vi "BTK Model_Janson.vi"(9 "V":dbl[](array[numeric])=[-0.1, -0.099, -0.098, -0.097, -0.096, -0.095, -0.094, -0.093, -0.092, -0.091, -0.09000000000000001, -0.08900000000000001, -0.08800000000000001, -0.08700000000000001, -0.08600000000000001, -0.085, -0.084, -0.083, -0.082, -0.081, -0.08, -0.079, -0.07800000000000001, -0.07700000000000001, -0.07600000000000001, -0.07500000000000001, -0.07400000000000001, -0.07300000000000001, -0.07200000000000001, -0.07100000000000001, -0.07, -0.069, -0.068, -0.067, -0.066, -0.065, -0.064, -0.063, -0.062000000000000006, -0.061000000000000006, -0.060000000000000005, -0.059000000000000004, -0.058, -0.057, -0.05600000000000001, -0.05500000000000001, -0.054000000000000006, -0.053000000000000005, -0.052000000000000005, -0.051000000000000004, -0.05, -0.049, -0.048, -0.04700000000000001, -0.046000000000000006, -0.045000000000000005, -0.044000000000000004, -0.043000000000000003, -0.042, -0.041, -0.04000000000000001, -0.03900000000000001, -0.038000000000000006, -0.037000000000000005, -0.036000000000000004, -0.035, -0.034, -0.033, -0.032, -0.031, -0.03, -0.028999999999999998, -0.027999999999999997, -0.02700000000000001, -0.02600000000000001, -0.02500000000000001, -0.024000000000000007, -0.023000000000000007, -0.022000000000000006, -0.021000000000000005, -0.020000000000000004, -0.019000000000000003, -0.018000000000000002, -0.017, -0.016, -0.015, -0.013999999999999999, -0.012999999999999998, -0.01200000000000001, -0.01100000000000001, -0.010000000000000009, -0.009000000000000008, -0.008000000000000007, -0.007000000000000006, -0.006000000000000005, -0.0050000000000000044, -0.0040000000000000036, -0.0030000000000000027, -0.0020000000000000018, -0.0010000000000000009, 0.0, 0.0010000000000000009, 0.0020000000000000018, 0.0030000000000000027, 0.0040000000000000036, 0.0049999999999999906, 0.0059999999999999915, 0.006999999999999992, 0.007999999999999993, 0.008999999999999994, 0.009999999999999995, 0.010999999999999996, 0.011999999999999997, 0.012999999999999998, 0.013999999999999999, 0.015, 0.016, 0.017, 0.018000000000000002, 0.019000000000000003, 0.01999999999999999, 0.02099999999999999, 0.021999999999999992, 0.022999999999999993, 0.023999999999999994, 0.024999999999999994, 0.025999999999999995, 0.026999999999999996, 0.027999999999999997, 0.028999999999999998, 0.03, 0.031, 0.032, 0.033, 0.034, 0.035, 0.036000000000000004, 0.037000000000000005, 0.038000000000000006, 0.03900000000000001, 0.04000000000000001, 0.04100000000000001, 0.04200000000000001, 0.04300000000000001, 0.04400000000000001, 0.044999999999999984, 0.045999999999999985, 0.046999999999999986, 0.04799999999999999, 0.04899999999999999, 0.04999999999999999, 0.05099999999999999, 0.05199999999999999, 0.05299999999999999, 0.05399999999999999, 0.05499999999999999, 0.055999999999999994, 0.056999999999999995, 0.057999999999999996, 0.059, 0.06, 0.061, 0.062, 0.063, 0.064, 0.065, 0.066, 0.067, 0.068, 0.069, 0.07, 0.07100000000000001, 0.07200000000000001, 0.07300000000000001, 0.07400000000000001, 0.07500000000000001, 0.07599999999999998, 0.07699999999999999, 0.07799999999999999, 0.07899999999999999, 0.07999999999999999, 0.08099999999999999, 0.08199999999999999, 0.08299999999999999, 0.08399999999999999, 0.08499999999999999, 0.086, 0.087, 0.088, 0.089, 0.09, 0.091, 0.092, 0.093, 0.094, 0.095, 0.096, 0.097, 0.098, 0.099, 0.1], 10 "Parameters":T1={"Gama"=0.001, "Delta"=0.03, "Z"=1.0, "P"=0.0, "T"=50.0, "Lower limit"=-10.0, "Upper limit"=10.0, "Resolution"=0.01} {"Resolution" format="%#_6peV"; "Upper limit" format="%#_6peV"; "Lower limit" format="%#_6peV"; "T" format="%#_6pK"; "Delta" format="%#_6peV"; "Gama" format="%#_6peV"}) -> (2 "Conductivity":dbl[](array[numeric]))   [LabVIEW 2021]
uses:
  Parameters.ctl
panel:
  in  "Normalize":bool
  out "1/x":dbl
  out "I-V":cluster{"Steps":dbl[], "dX/dt":dbl[]}(graph)
  out "f(E-eV)-f(E)":cluster{"Steps":dbl[], "dX/dt":dbl[]}(graph)
  out "Z":cluster{"Steps":dbl[], "dX/dt":dbl[]}(graph)
  out "dIdV":cluster{"Steps":dbl[], "dX/dt":dbl[]}(graph)
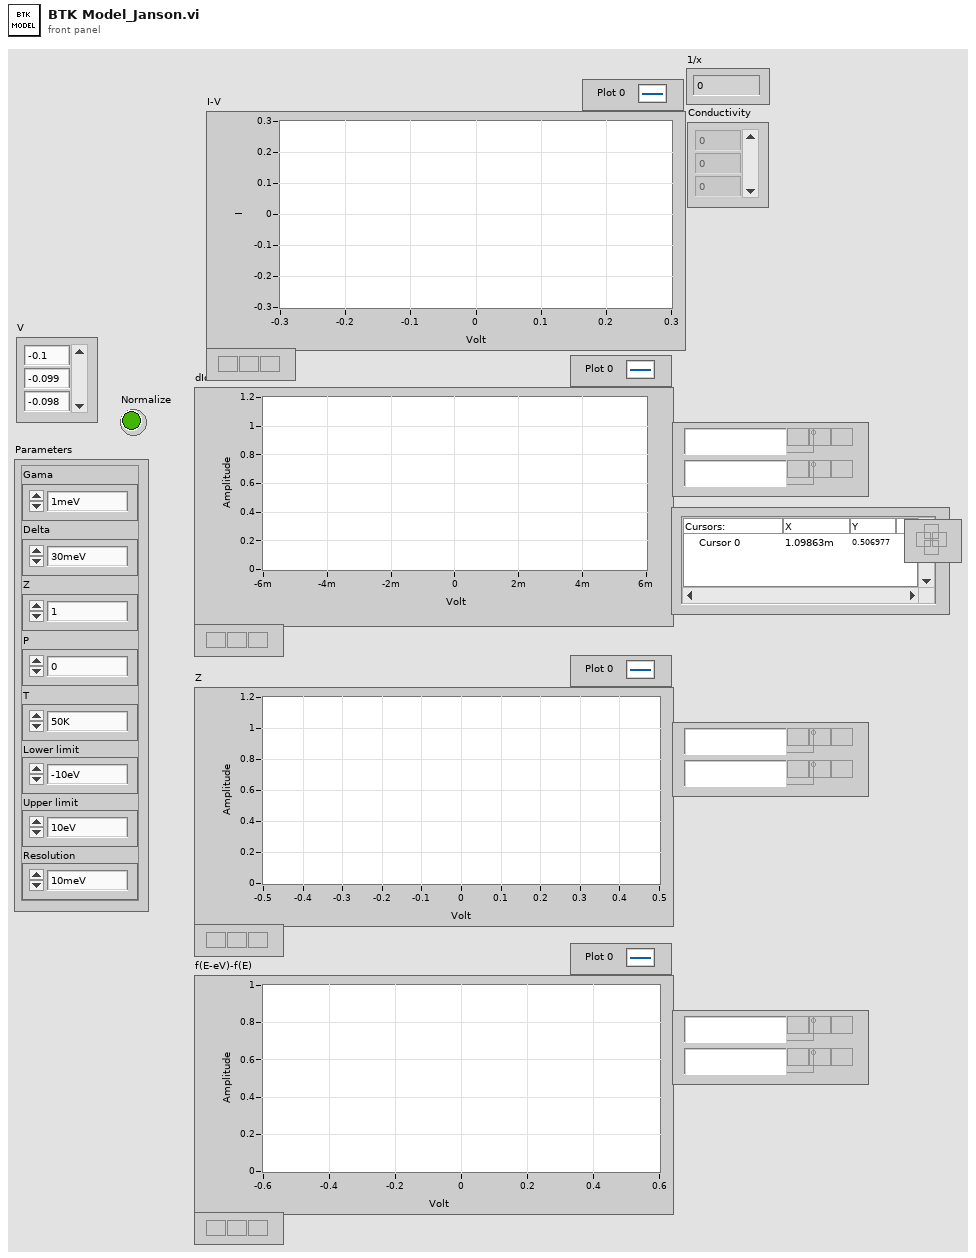
[diagram p1: front panel]
types:
  T1 = typedef "Parameters.ctl" = cluster{"Gama":dbl, "Delta":dbl, "Z":dbl, "P":dbl, "T":dbl, "Lower limit":dbl, "Upper limit":dbl, "Resolution":dbl}
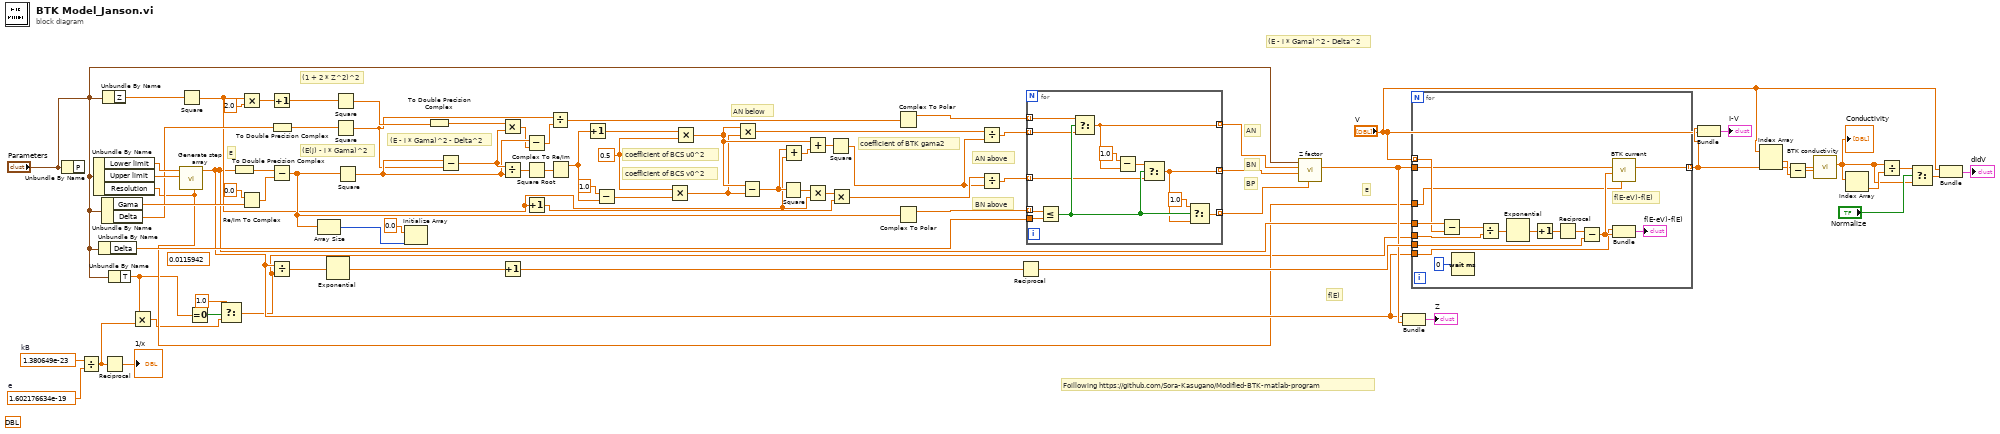
[diagram p0: block diagram]
diagram:
  w19 = 1.602176634e-19  # e
  (unwired) ext[unit] 1.602176634e-19
  w20 = 1.380649e-23  # kB
  (unwired) 0.0115942
  w66 = 0.5
  # "f(E)"
  # "E"
  # "BP"
  # "BN"
  # "AN"
  # "Foillowing https://github.com/Sora-Kasugano/Modified-BTK-matlab-program"
  # "BN above"
  # "AN above"
  # "AN below"
  # "(E(j) - i * Gama)^2"
  # "(E - i * Gama)^2 - Delta^2"
  # "(1 + 2 * Z^2)^2"
  # "E"
  # "(E - i * Gama)^2 - Delta^2"
  # "coefficient of BTK gama2"
  # "coefficient of BCS v0^2"
  # "coefficient of BCS u0^2"
  n1 = Unbundle By Name("Parameters") -> ()  [unwired: 1 out]
  n2 = Divide(x=w20, y=w19) -> (x/y=w7:dbl)
  n3 = Unbundle By Name("Parameters") -> ("Lower limit"=w80:dbl, "Upper limit"=w79:dbl, "Resolution"=w14:dbl)
  n4 = Unbundle By Name("Parameters") -> ("Delta"=w37:dbl)
  n5 = Unbundle By Name("Parameters") -> ("Gama"=w77:dbl, "Delta"=w74:dbl)
  n6 = Unbundle By Name("Parameters") -> ("Z"=w65:dbl)
  n7 = Reciprocal(x=w7) -> (1/x=→"1/x":dbl)
  n8 = Unbundle By Name("Parameters") -> ("T"=w6:dbl)
  n9 = Multiply(x=w6, y=w7) -> (x*y=w8:dbl)
  n10 = call "Generate step array.vi"("Step"=w14, "End"=w79, "Start"=w80) -> ("Steps"=w22:dbl[])  [unwired: 8 in]
  n11 = Square(x=w65) -> (x^2=w43:dbl)
  n12 = Equal To 0?(x=w6) -> (x = 0?=w11:bool)
  n13 = Select(t=1.0, s=w11, f=w8) -> (s? t:f=w9:dbl)
  n14 = To Double Precision Complex(1:w22) -> (0:w76:cdb[])
  n15 = Multiply(x=w43, y=2.0) -> (x*y=w59:dbl)
  n16 = Re/Im To Complex(1:w77, 2:0.0) -> (0:w75:cdb)
  n17 = Increment(x=w59) -> (x+1=w58:dbl)
  n18 = Subtract(x=w76, y=w75) -> (x-y=w46:cdb[])
  n19 = Divide(x=w22, y=w9) -> (x/y=w33:dbl[])
  n20 = To Double Precision Complex(1:w74) -> (0:w73:cdb)
  n21 = Array Size(array=w46) -> (size(s)=w61:i32)
  n22 = Exponential(1:w33) -> (0:w32:dbl[])
  n23 = Square(x=w58) -> (x^2=w57:dbl)
  n24 = Square(x=w73) -> (x^2=w51:cdb)
  n25 = Square(x=w46) -> (x^2=w54:cdb[])
  n26 = Initialize Array(0.0, w61) -> ()  [unwired: 1 out]
  n27 = To Double Precision Complex(1:w57) -> (0:w55:cdb)
  n28 = Subtract(x=w54, y=w51) -> (x-y=w56:cdb[])
  n29 = Multiply(x=w55, y=w56) -> (x*y=w53:cdb[])
  n30 = Divide(x=w56, y=w54) -> (x/y=w72:cdb[])
  n31 = Increment(x=w32) -> (x+1=w31:dbl[])
  n32 = Subtract(x=w54, y=w53) -> (x-y=w52:cdb[])
  n33 = Square Root(x=w72) -> (sqrt(x)=w71:cdb[])
  n34 = Increment(x=w43) -> (x+1=w41:dbl)
  n35 = Divide(x=w51, y=w52) -> (x/y=w47:cdb[])
  n36 = Complex To Re/Im(x + iy=w71) -> (x=w69:dbl[])  [unwired: 1 out]
  n37 = Increment(x=w69) -> (x+1=w70:dbl[])
  n38 = Subtract(x=1.0, y=w69) -> (x-y=w67:dbl[])
  n39 = Multiply(x=w66, y=w67) -> (x*y=w49:dbl[])
  n40 = Multiply(x=w70, y=w66) -> (x*y=w50:dbl[])
  n41 = Multiply(x=w50, y=w49) -> (x*y=w48:dbl[])
  n42 = Subtract(x=w50, y=w49) -> (x-y=w45:dbl[])
  n43 = Square(x=w45) -> (x^2=w44:dbl[])
  n44 = Add(x=w45, y=w43) -> (x+y=w64:dbl[])
  n45 = Add(x=w50, y=w64) -> (x+y=w63:dbl[])
  n46 = Multiply(x=w44, y=w43) -> (x*y=w42:dbl[])
  n47 = Square(x=w63) -> (x^2=w39:dbl[])
  n48 = Multiply(x=w42, y=w41) -> (x*y=w40:dbl[])
  n49 = Complex To Polar(r * e^(i*theta)=w47) -> (r=w36:dbl[])  [unwired: 1 out]
  n50 = Complex To Polar(r * e^(i*theta)=w46) -> (r=w38:dbl[])  [unwired: 1 out]
  n51 = Divide(x=w48, y=w39) -> (x/y=w34:dbl[])
  n52 = Divide(x=w40, y=w39) -> (x/y=w35:dbl[])
  n53 = Reciprocal(x=w31) -> (1/x=w30:dbl[])
  n54 = for {
    tunnel: w38 -> [w87] mode=indexing
    tunnel: w37 -> [w88]
    tunnel: w36 -> [w86] mode=indexing
    tunnel: w35 -> [w85] mode=indexing
    tunnel: w34 -> [w84] mode=indexing
    tunnel: [w83] -> w28 mode=indexing
    tunnel: [w82] -> w27 mode=indexing
    tunnel: [w81] -> w26 mode=indexing
    n55 = Less Or Equal?(x=w87, y=w88) -> (x <= y?=w89:bool)
    n56 = Select(t=w86, s=w89, f=w84) -> (s? t:f=w83:dbl)
    n57 = Subtract(x=1.0, y=w83) -> (x-y=w92:dbl)
    n58 = Select(t=w92, s=w89, f=w85) -> (s? t:f=w82:dbl)
    n59 = Select(t=1.0, s=w89, f=w82) -> (s? t:f=w81:dbl)
  }
  n60 = call "Z factor.vi"("BP"=w26, "BN"=w27, "AN"=w28, "Parameters"="Parameters") -> ("z factor"=w24:dbl[])  [unwired: 7 in]
  n61 = Bundle("Steps"=w22, "z factor"=w24) -> (→"Z":cluster{"Steps":dbl[], "z factor":dbl[]})  [unwired: 1 in]
  n62 = for {
    tunnel: "V" -> [w107] mode=indexing
    tunnel: w22 -> [w108]
    tunnel: w9 -> [w104]
    tunnel: w30 -> [w102]
    tunnel: w24 -> [w99]
    tunnel: [w98] -> w13 mode=indexing
    tunnel: w22 -> [w94]
    tunnel: w14 -> [w93]
    # "f(E-eV)-f(E)"
    n63 = Subtract(x=w108, y=w107) -> (x-y=w106:dbl[])
    n64 = Wait (ms)(milliseconds to wait=u32 0) -> ()  [unwired: 1 out]
    n65 = Divide(x=w106, y=w104) -> (x/y=w105:dbl[])
    n66 = Exponential(1:w105) -> (0:w103:dbl[])
    n67 = Increment(x=w103) -> (x+1=w101:dbl[])
    n68 = Reciprocal(x=w101) -> (1/x=w100:dbl[])
    n69 = Subtract(x=w100, y=w102) -> (x-y=w97:dbl[])
    n70 = call "BTK current.vi"("dx"=w93, "f factor"=w97, "z factor"=w99) -> ("I current"=w98:dbl)  [unwired: 8 in]
    n71 = Bundle("Steps"=w94, w97) -> (→"f(E-eV)-f(E)":cluster{"Steps":dbl[], dbl[]})  [unwired: 1 in]
  }
  n72 = Bundle(w13, "V"="V") -> (→"I-V":cluster{dbl[], "V":dbl[]})  [unwired: 1 in]
  n73 = Index Array(array="V") -> (element #1=w17:dbl, element #2=w16:dbl)  [unwired: 2 in]
  n74 = Subtract(x=w16, y=w17) -> (x-y=w15:dbl)
  n75 = call "BTK conductivity.vi"("dx"=w15, "Current"=w13) -> ("Conductivity"=w2:dbl[])  [unwired: 8 in, 1 out]
  "Conductivity" <- w2
  n76 = Index Array(array=w2) -> (element=w5:dbl)  [unwired: 1 in]
  n77 = Divide(x=w2, y=w5) -> (x/y=w4:dbl[])
  n78 = Select(t=w4, s="Normalize", f=w2) -> (s? t:f=w1:dbl[])
  n79 = Bundle("V"="V", "Conductivity"=w1) -> (→"dIdV":cluster{"V":dbl[], "Conductivity":dbl[]})  [unwired: 1 in]
